vi "Results_file_header.vi"() -> (0 "Header":string)   [LabVIEW 2011]
uses:
  Controls/Post_Process.ctl
  Globals/Meas_global.vi
panel:
  # "Create file Header"
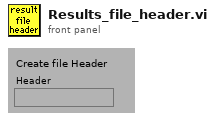
[diagram p1: front panel]
types:
  T1 = typedef "Post_Process.ctl" = enum16{"Take New Data", "Post Process Raw Data File"}
  T2 = typedef "Ch_and_Spans.ctl" = cluster{"high limit (10V)":sgl, "low limit (-10V)":sgl, "Ch No":i16, "Var name":string, "Use Latest Calib":bool}
  T3 = typedef "Board_Types.ctl" = enum16{"Simulate", "Local ADAM", "Server ADAM", "NI-DAQmx", "NI-DAQmxBase", "ADC488", "DT LV-link"}
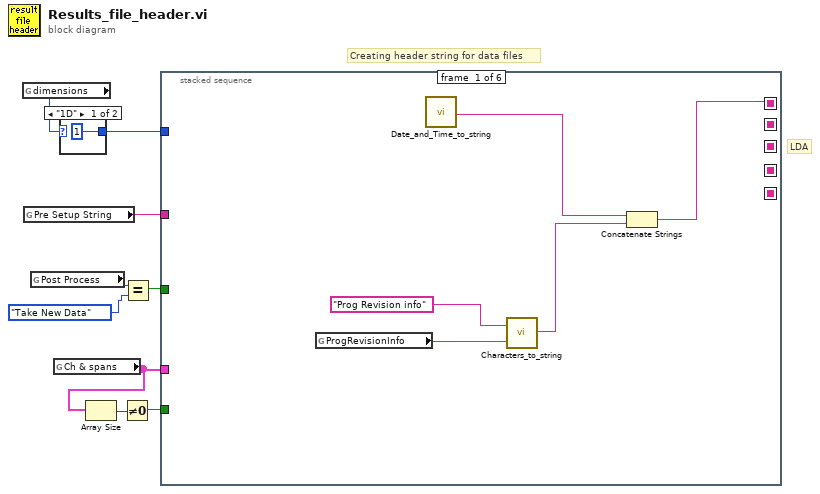
[diagram p0: block diagram]
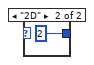
[diagram p2: hidden frame]
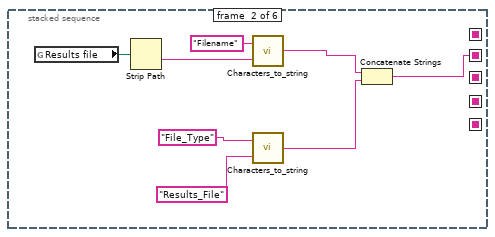
[diagram p3: hidden frame]
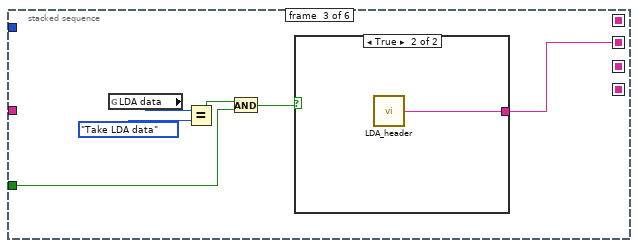
[diagram p4: hidden frame]
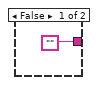
[diagram p5: hidden frame]
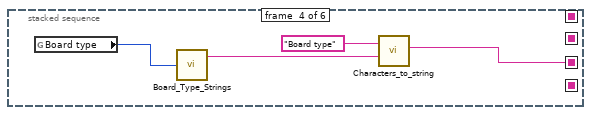
[diagram p6: hidden frame]
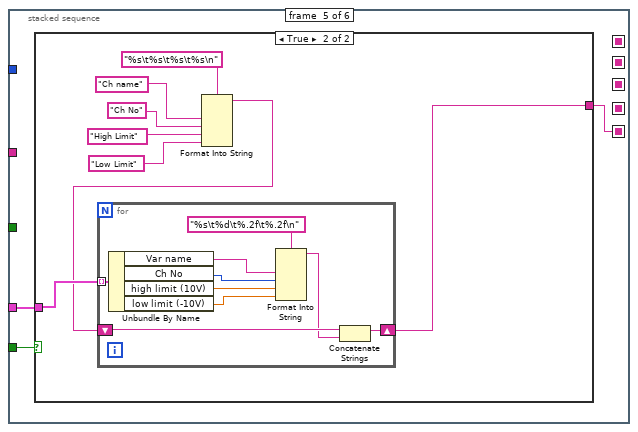
[diagram p7: hidden frame]
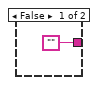
[diagram p8: hidden frame]
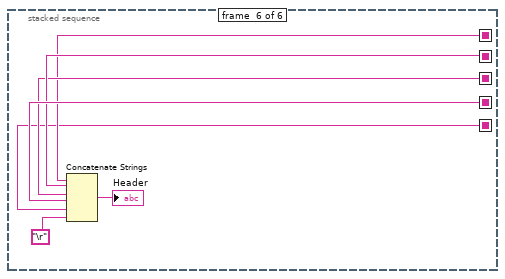
[diagram p9: hidden frame]
diagram:
  # "LDA"
  # "Creating header string for data files"
  n1 = global read "Meas_global.vi" "dimensions"() -> (w9:enum16{"1D", "2D"})
  n2 = global read "Meas_global.vi" "Pre Setup String"() -> (w2:string)
  n3 = global read "Meas_global.vi" "Post Process"() -> (w7:T1)
  n4 = global read "Meas_global.vi" "Ch & spans"() -> (w4:T2[])
  n5 = case shown="\"1D\"" w9 {
    tunnel: [1 2] -> w8
    frame "1D" {
    }
    frame "2D" {
    }
  }
  n6 = Array Size(array=w4) -> (size(s)=w5:i32)
  n7 = Not Equal To 0?(x=w5) -> (x != 0?=w3:bool)
  n8 = Equal?(x=w7, y=Post_Process."Take New Data" ("Post Process")) -> (x = y?=w6:bool)
  n9 = stacked-sequence {
    seq-local: [_ _ _ w33 _ _] -> [_ _ _ _ _ w64]
    seq-local: [_ w17 _ _ _ _] -> [_ _ _ _ _ w63]
    seq-local: [_ _ w26 _ _ _] -> [_ _ _ _ _ w62]
    seq-local: [w13 _ _ _ _ _] -> [_ _ _ _ _ w60]
    seq-local: [_ _ _ _ w37 _] -> [_ _ _ _ _ w59]
    tunnel: w8 -> [_ _ _ _ _ _]
    tunnel: w6 -> [_ _ w25 _ _ _]
    tunnel: w4 -> [_ _ _ _ w38 _]
    tunnel: w3 -> [_ _ _ _ w39 _]
    tunnel: w2 -> [_ _ _ _ _ _]
    frame #0 {
      n10 = global read "Meas_global.vi" "ProgRevisionInfo"() -> (w12:string)
      n11 = call "Date_and_Time_to_string.vi"() -> ("Date and time (spreadsheet)"=w14:string)
      n12 = call "Characters_to_string.vi"("Characters to write"=w12, "Label for characters"="Prog Revision info") -> ("Output string"=w15:string)
      n13 = Concatenate Strings(w14, w15) -> (w13:string)
    }
    frame #1 {
      n14 = global read "Meas_global.vi" "Results file"() -> (w23:path)
      n15 = Strip Path(path=w23) -> (name=w22:string)  [unwired: 1 out]
      n16 = call "Characters_to_string.vi"("Characters to write"=w22, "Label for characters"="Filename") -> ("Output string"=w19:string)
      n17 = call "Characters_to_string.vi"("Characters to write"="Results_File", "Label for characters"="File_Type") -> ("Output string"=w18:string)
      n18 = Concatenate Strings(w19, w18) -> (w17:string)
    }
    frame #2 {
      n19 = global read "Meas_global.vi" "LDA data"() -> (w28:enum16{"No LDA data", "Take LDA data"})
      n20 = Equal?(x=w28, y=enum16{"No LDA data", "Take LDA data"}."Take LDA data" ("LDA data")) -> (x = y?=w30:bool)
      n21 = And(x=w30, y=w25) -> (x .and. y?=w27:bool)
      n22 = case shown="True" w27 {
        tunnel: ["" w32] -> w26
        frame False {
        }
        frame True {
          n23 = call "LDA_header.vi"() -> ("LDA Header string"=w32:string)  [unwired: 3 out]
        }
      }
    }
    frame #3 {
      n24 = global read "Meas_global.vi" "Board type"() -> (w34:T3)
      n25 = call "Board_Type_Strings.vi"("Board type"=w34) -> ("Board String"=w35:string)  [unwired: 1 out]
      n26 = call "Characters_to_string.vi"("Characters to write"=w35, "Label for characters"="Board type") -> ("Output string"=w33:string)
    }
    frame #4 {
      n27 = case shown="True" w39 {
        tunnel: w38 -> [_ w43]
        tunnel: ["" w41] -> w37
        frame False {
        }
        frame True {
          n28 = Format Into String(format string="%s\t%s\t%s\t%s\n" ("Format String"), "Ch name", "Ch No", "High Limit", "Low Limit") -> (resulting string=w42:string)  [unwired: 2 in, 1 out]
          n29 = for {
            tunnel: w43 -> [w57] mode=indexing
            shift-right: [w49] -> w41
            shift-left: w42 -> [w51]
            n30 = Unbundle By Name(w57) -> ("Var name"=w56:string, "Ch No"=w55:i16, "high limit (10V)"=w54:sgl, "low limit (-10V)"=w53:sgl)
            n31 = Format Into String(format string="%s\t%d\t%.2f\t%.2f\n" ("Format String"), w56, w55, w54, w53) -> (resulting string=w50:string)  [unwired: 2 in, 1 out]
            n32 = Concatenate Strings(w51, w50) -> (w49:string)
          }
        }
      }
    }
    frame #5 {
      n33 = Concatenate Strings(w60, w63, w62, w64, w59, "\r") -> (→"Header":string)
    }
  }
